vi "Calculate Calibrated Resistance.vi"(3 "Waveform Array - UnBiased":waveform(dbl)[](array[waveform]), 4 "Waveform Array - Biased":waveform(dbl)[](array[waveform]), 5 "SMU_Current":dbl=0.005) -> (1 "DC Offset":dbl, 2 "Resistance":dbl)   [LabVIEW 2010]
uses:
  <vilib>/Analysis/NI_AALBase.lvlib
panel:
  out "Biased":waveform(dbl)[](graph)
  out "UnBiased":waveform(dbl)[](graph)
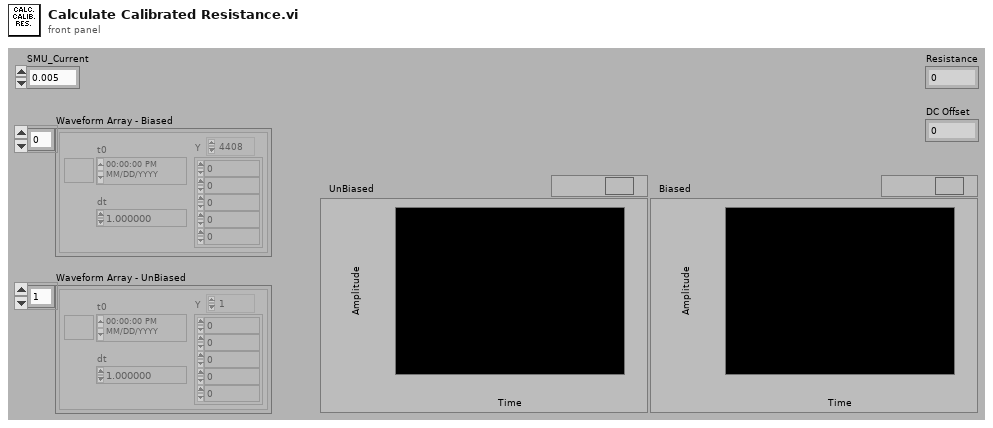
[diagram p1: front panel]
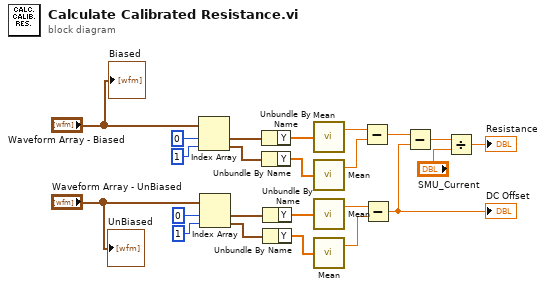
[diagram p0: block diagram]
diagram:
  n1 = Index Array(array="Waveform Array - Biased", index #1=0 ("index"), index #2=1 ("index")) -> (element #1=w19:waveform(dbl), element #2=w21:waveform(dbl))
  n2 = Index Array(array="Waveform Array - UnBiased", index #1=0 ("index"), index #2=1 ("index")) -> (element #1=w14:waveform(dbl), element #2=w15:waveform(dbl))
  n3 = Unbundle By Name(w19) -> ("Y"=w9:dbl[])
  n4 = Unbundle By Name(w21) -> ("Y"=w10:dbl[])
  n5 = Unbundle By Name(w14) -> ("Y"=w11:dbl[])
  n6 = Unbundle By Name(w15) -> ("Y"=w12:dbl[])
  n7 = call <vilib>:"Mean.vi"("X"=w9) -> ("mean"=w8:dbl)  [unwired: 1 out]
  n8 = call <vilib>:"Mean.vi"("X"=w10) -> ("mean"=w7:dbl)  [unwired: 1 out]
  n9 = call <vilib>:"Mean.vi"("X"=w11) -> ("mean"=w6:dbl)  [unwired: 1 out]
  n10 = call <vilib>:"Mean.vi"("X"=w12) -> ("mean"=w5:dbl)  [unwired: 1 out]
  n11 = Subtract(x=w8, y=w7) -> (x-y=w4:dbl)
  n12 = Subtract(x=w6, y=w5) -> (x-y=w3:dbl)
  "DC Offset" <- w3
  n13 = Subtract(x=w4, y=w3) -> (x-y=w13:dbl)
  n14 = Divide(x=w13, y="SMU_Current") -> (x/y=→"Resistance":dbl)
  "UnBiased" <- "Waveform Array - UnBiased"
  "Biased" <- "Waveform Array - Biased"
